vi "Initialize.vi"(8 "Error In (No Error)":errorcluster, 10 "General Settings:Timeout Value":u32=9000, 11 "RS232 Port In":refnum<visa-resource-name>) -> (0 "Error Out":errorcluster, 3 "RS232 Port Out":refnum<visa-resource-name>)   [LabVIEW 2016, in "SDI-12.lvlib"]
doc: "Configures and starts a VISA session with the RS232 to SDI-12 converter."
uses:
  SDI-12.lvlib
panel:
  # "(c) 2008 National Instruments.  ALL RIGHTS RESERVED."
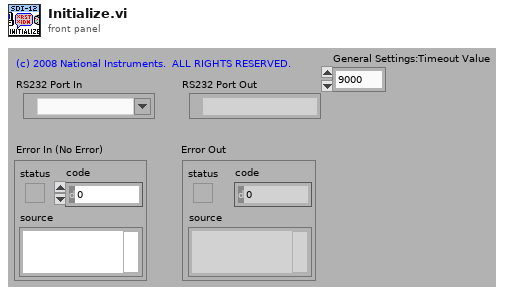
[diagram p1: front panel]
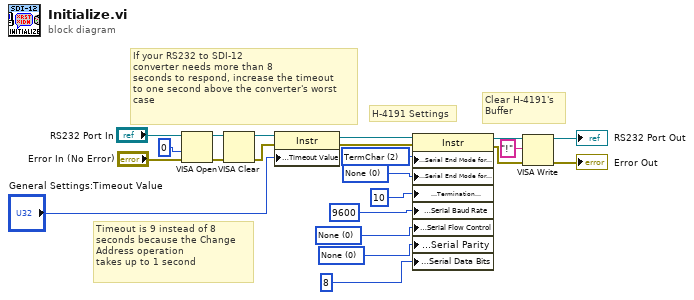
[diagram p0: block diagram]
diagram:
  w6 = u16 0 items=["None", "Odd", "Even", "Mark", "Space"] ("Serial Settings:Parity")
  w7 = u16 0 items=["None", "XON/XOFF", "RTS/CTS", "XON/XOFF & RTS/CTS", "DTR/DSR", "XON/XOFF & DTR/DSR"] ("Serial Settings:Flow Control")
  w10 = u16 0 items=["None", "Last Bit", "TermChar", "Break"] ("Serial Settings:End Mode for Writes")
  w11 = u16 2 items=["None", "LastBit", "TermChar"] ("Serial Settings:Serial End Mode for Reads")
  # "Timeout is 9 instead of 8\nseconds because the Change \nAddress operation\ntakes up to 1 second"
  # "If your RS232 to SDI-12\nconverter needs more than 8\nseconds to respond, increase the timeout\nto one second above the converter's worst\ncase"
  # "Clear H-4191's \nBuffer"
  # "H-4191 Settings"
  n1 = VISA Open(access mode=u32 0, error in (no error)="Error In (No Error)", VISA resource name="RS232 Port In") -> (VISA resource name=w17:refnum<visa-resource-name>, error out=w16:errorcluster)  [unwired: 2 in]
  n2 = VISA Clear(VISA resource name=w17, error in (no error)=w16) -> (VISA resource name out=w15:refnum<visa-resource-name>, error out=w14:errorcluster)
  n3 = property class="Instr"(reference=w15, error in=w14, "General Settings:Timeout Value"="General Settings:Timeout Value") -> (reference out=w20:refnum<visa-resource-name>, error out=w19:errorcluster)
  n4 = property class="Instr"(reference=w20, error in=w19, "Serial Settings:Serial End Mode for Reads"=w11, "Serial Settings:Serial End Mode for Writes"=w10, "Message Based Settings:Termination Character"=u8 10, "Serial Settings:Serial Baud Rate"=u32 9600 ("Serial Settings:Baud Rate"), "Serial Settings:Serial Flow Control"=w7, "Serial Settings:Serial Parity"=w6, "Serial Settings:Serial Data Bits"=u16 8 ("Serial Settings:Data Bits")) -> (reference out=w1:refnum<visa-resource-name>, error out=w2:errorcluster)
  n5 = VISA Write(VISA resource name=w1, write buffer="!", error in (no error)=w2) -> (VISA resource name out=→"RS232 Port Out":refnum<visa-resource-name>, error out=→"Error Out":errorcluster)  [unwired: 1 out]
